vi "xcite.vi"(8 "error in (no error)":errorcluster, 11 "Xcite in":refnum<class "Xcite.lvclass">) -> (0 "error out":errorcluster, 2 "xcite":u64, 3 "Xcite out":refnum<class "Xcite.lvclass">)   [LabVIEW 2019, in "Xcite.lvclass"]
doc: "Returns the handle to the XCite device associated wth this object. The handle can be used with low-level XCitefunctions."
uses:
  Xcite.lvclass
  Xcite.lvclass/Xcite.ctl
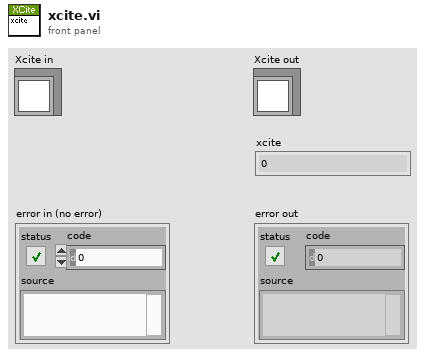
[diagram p1: front panel]
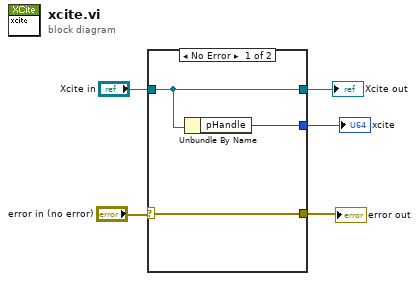
[diagram p0: block diagram]
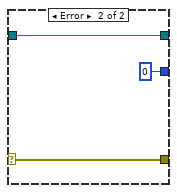
[diagram p2: hidden frame]
diagram:
  n1 = case shown="No Error" "error in (no error)" {
    selector: "error in (no error)" -> [w6 w11]
    tunnel: "Xcite in" -> [w7 w10]
    tunnel: [w8 u64 0 ("pHandle")] -> w1
    tunnel: [w7 w10] -> w4
    tunnel: [w6 w11] -> w2
    frame No Error {
      n2 = Unbundle By Name(w7) -> ("pHandle"=w8:u64)
    }
    frame Error {
    }
  }
  "Xcite out" <- w4
  "error out" <- w2
  "xcite" <- w1
